vi "D_bank_control_command_parallel.vi"(0 "SI804.lvclass in":refnum<class "SI804.lvclass">, 5 "3 JSA30 DG101\nXA01":bool, 7 "3 JSA20 DT303\nXA01":bool, 11 "error in":errorcluster) -> (4 "SI804.lvclass out":refnum<class "SI804.lvclass">, 6 "D-bank Ctrl M/A":bool, 8 "D-quads par":bool, 15 "error out":errorcluster)   [LabVIEW 2022 SP3, in "SI804.lvclass"]
uses:
  SI804.lvclass
  SI804.lvclass/SI804.ctl
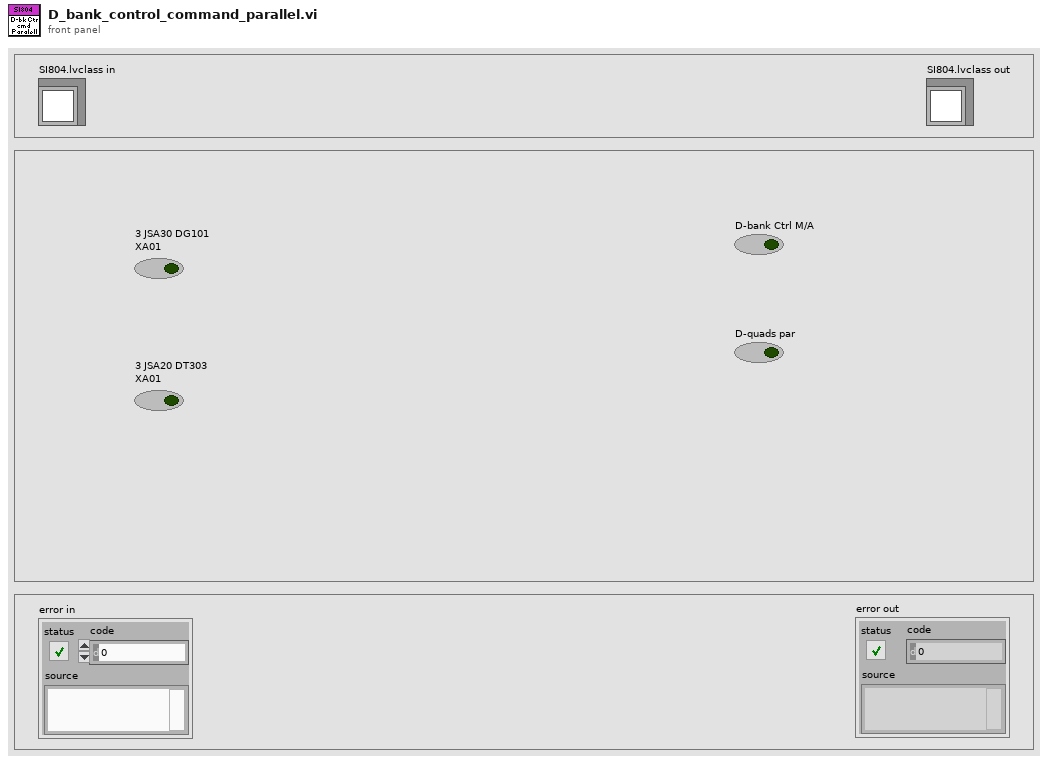
[diagram p1: front panel]
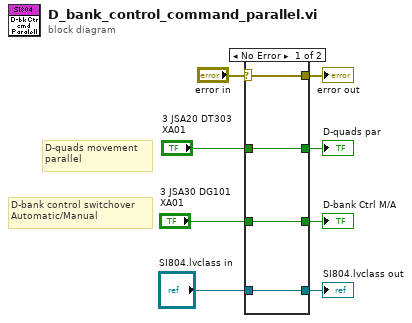
[diagram p0: block diagram]
diagram:
  # "D-quads movement\nparallel"
  # "D-bank control switchover\nAutomatic/Manual"
  n1 = case shown="No Error" "error in" {
    selector: "error in" -> [w10 w13]
    tunnel: "3 JSA30 DG101\nXA01" -> [w12 _]
    tunnel: "3 JSA20 DT303\nXA01" -> [w11 _]
    tunnel: "SI804.lvclass in" -> [w9 w14]
    tunnel: [w12 _] -> w4
    tunnel: [w11 _] -> w3
    tunnel: [w10 w13] -> w2
    tunnel: [w9 w14] -> w1
    frame No Error {
    }
    frame Error {
    }
  }
  "D-bank Ctrl M/A" <- w4
  "D-quads par" <- w3
  "error out" <- w2
  "SI804.lvclass out" <- w1
